vi "T1_Pulse_CommandSTR_gen.vi"(0 "T1 Pulse Sequence":T2={"Preliminary Settings"={"Nº of Scans (ns)"=3, "Pulse Frequency"=10000000.0, "Nº of Vd"=3}, "Pulse Settings"={"Duration Signal P2"=20.0, "Power Level P2"=1023, "Phase P2"=90, "P2 Unit"=0, "Duration Signal P1"=20.0, "Power Level P1"=1023, "Phase P1"=90, "P1 Unit"=0}, "Acquisition Settings"={"Number Samples"=2000, "Time Between Points"=0.0, "Unit"=0}, "Delay Settings"={"Delay d1"=10.0, "Delay d2"=0.0, "d1 Unit"=0, "d2 Unit"=0, "Delay d30"=0.0, "d30 Unit"=0, "Vd Unit"=0, "Vd Values"="1"}} {"Delay Settings"."Vd Unit" items=["us", "ms"]; "Delay Settings"."d30 Unit" items=["us", "ms"]; "Delay Settings"."Delay d30" min=0.0 step=1.0; "Delay Settings"."d2 Unit" items=["us", "ms"]; "Delay Settings"."d1 Unit" items=["us", "ms"]; "Delay Settings"."Delay d2" min=0.0 step=1.0 format="%#_4g"; "Delay Settings"."Delay d1" min=0.0 step=1.0 format="%#_4g"; "Acquisition Settings"."Unit" items=["us", "ms"]; "Acquisition Settings"."Time Between Points" min=0.0 step=1.0; "Acquisition Settings"."Number Samples" step=1; "Pulse Settings"."P1 Unit" items=["us", "ms"]; "Pulse Settings"."Phase P1" max=270 step=90; "Pulse Settings"."Power Level P1" max=1023 step=1; "Pulse Settings"."Duration Signal P1" min=0.0 step=1.0 format="%#_4g"; "Pulse Settings"."P2 Unit" items=["us", "ms"]; "Pulse Settings"."Phase P2" max=270 step=90; "Pulse Settings"."Power Level P2" max=1023 step=1; "Pulse Settings"."Duration Signal P2" min=0.0 step=1.0 format="%#_4g"; "Preliminary Settings"."Nº of Vd" step=1; "Preliminary Settings"."Pulse Frequency" min=1.0 max=200000000.0 step=1000000.0 format="%^#_6e"; "Preliminary Settings"."Nº of Scans (ns)" step=1}, 5 "Manual Vd":dbl[](array[numeric])=[10.0, 340.0, 670.0, 1000.0] min=1.0 step=1.0) -> (4 "Array":string[](array[string]), 6 "T1 set times":T1={"Real Time P1"=20.011287076734621636, "Real Time P2"=20.011287076734621636, "Real Time d1"=10.036661125207804438, "Real Time d2"=1.462, "Real Time d30"=1.462, "Real Time AQS"=0.73746299999999999998}, 12 "Values Vd Used":dbl[](array[numeric]))   [LabVIEW 2011]
uses:
  Controls/Full_T1 Degree Pulse Settings.ctl
  Controls/T1_Preliminary Settings.ctl
  Controls/T1_Pulse Settings.ctl
  Controls/Acquisition Settings.ctl
  Controls/T1_Delay Settings.ctl
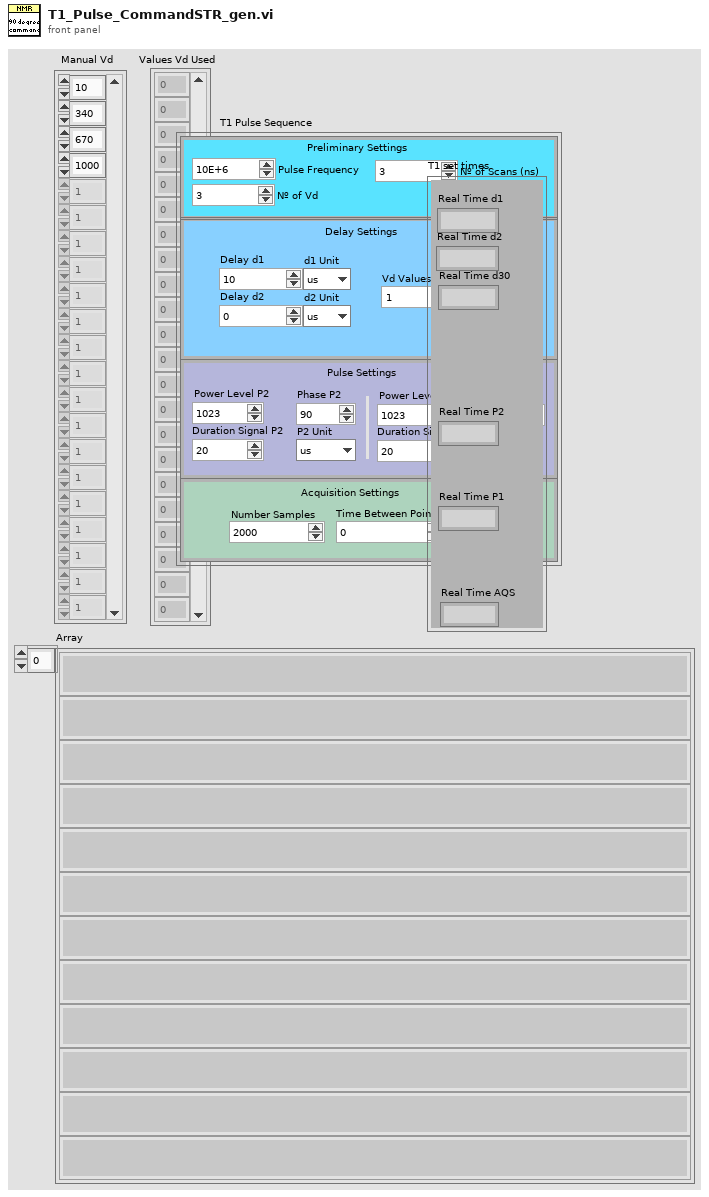
[diagram p1: front panel]
types:
  T1 = cluster{"Real Time P1":ext, "Real Time P2":ext, "Real Time d1":ext, "Real Time d2":ext, "Real Time d30":ext, "Real Time AQS":ext}
  T2 = typedef "Full_T1 Degree Pulse Settings.ctl" = cluster{"Preliminary Settings":T3, "Pulse Settings":T4, "Acquisition Settings":T5, "Delay Settings":T6}
  T3 = typedef "T1_Preliminary Settings.ctl" = cluster{"Nº of Scans (ns)":u16, "Pulse Frequency":dbl, "Nº of Vd":u16}
  T4 = typedef "T1_Pulse Settings.ctl" = cluster{"Duration Signal P2":dbl, "Power Level P2":u16, "Phase P2":u16, "P2 Unit":u8, "Duration Signal P1":dbl, "Power Level P1":u16, "Phase P1":u16, "P1 Unit":u8}
  T5 = typedef "Acquisition Settings.ctl" = cluster{"Number Samples":u16, "Time Between Points":dbl, "Unit":u8}
  T6 = typedef "T1_Delay Settings.ctl" = cluster{"Delay d1":dbl, "Delay d2":dbl, "d1 Unit":u8, "d2 Unit":u8, "Delay d30":dbl, "d30 Unit":u8, "Vd Unit":u8, "Vd Values":string}
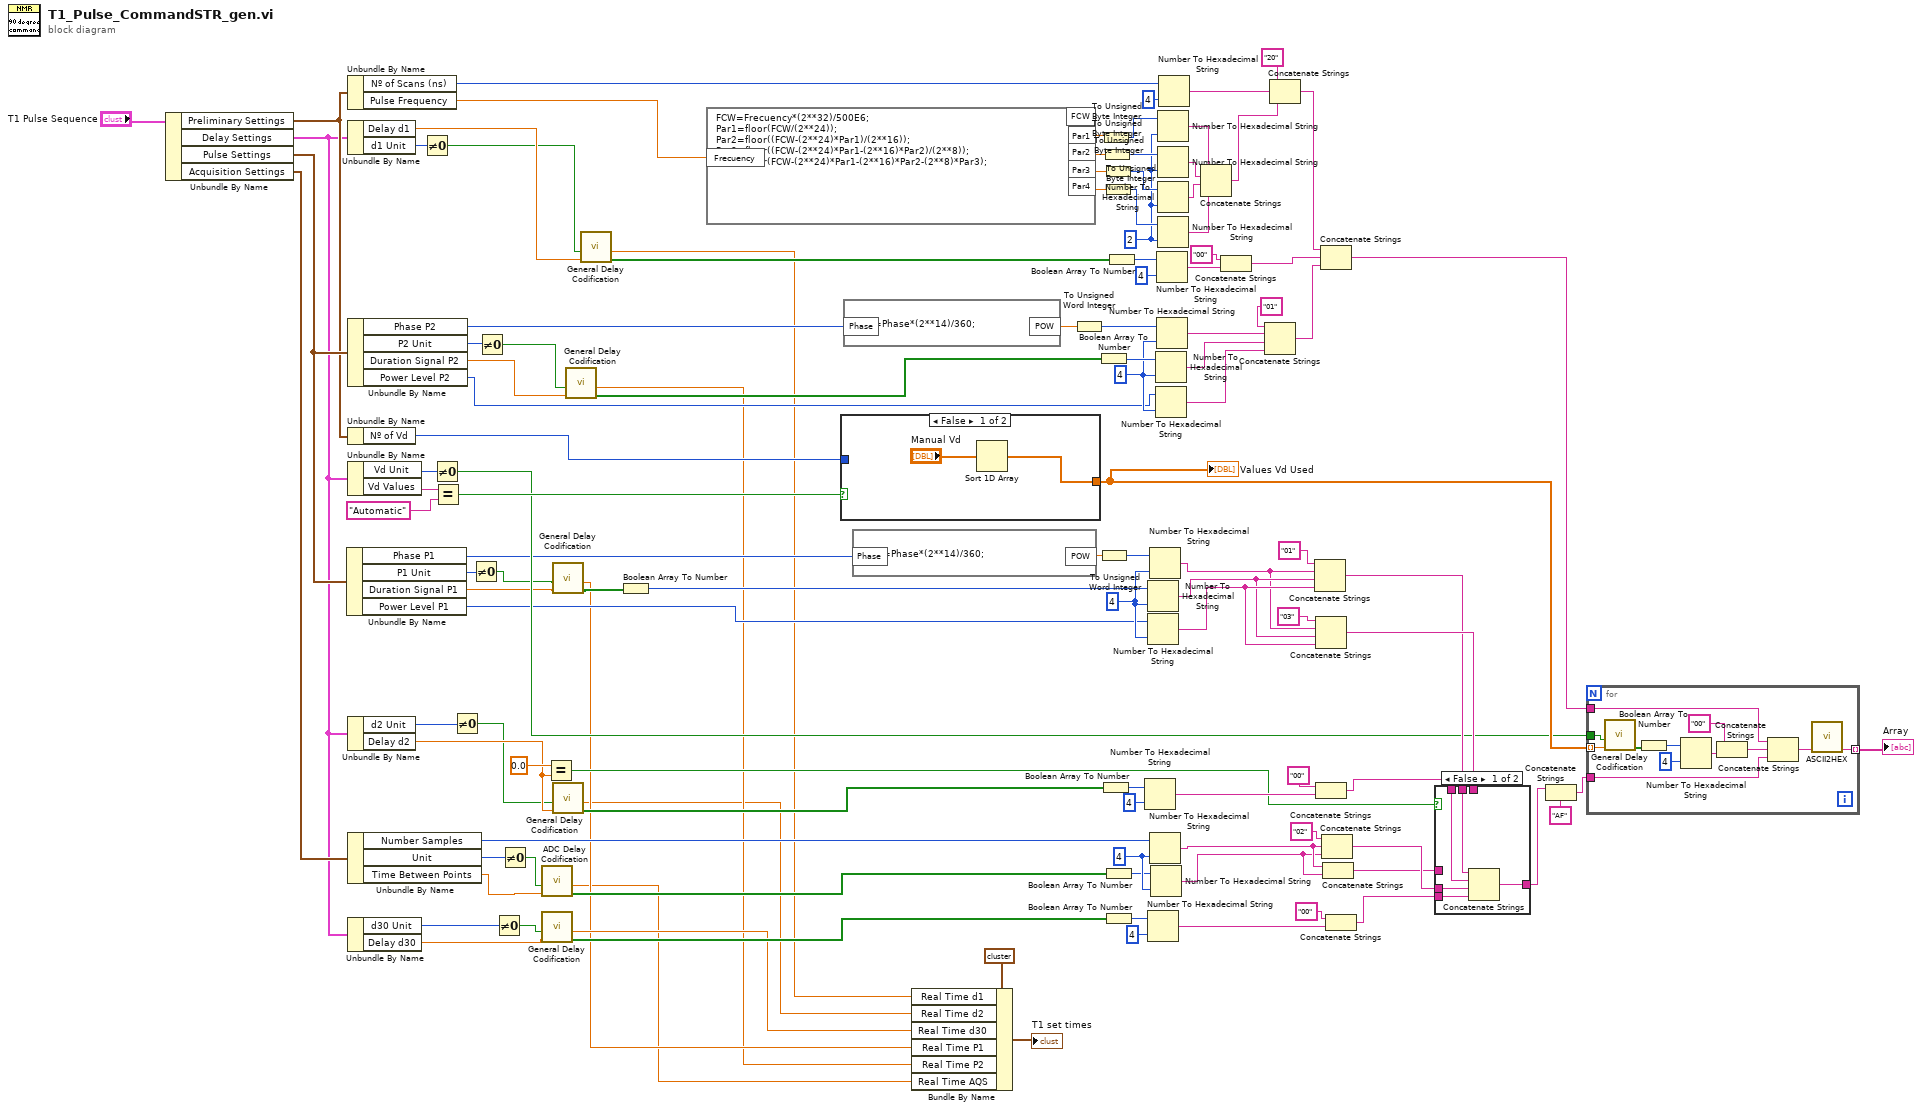
[diagram p0: block diagram]
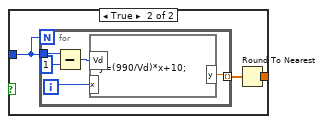
[diagram p2: hidden frame]
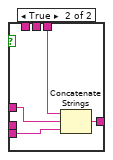
[diagram p3: hidden frame]
diagram:
  w78 = i16 2 ("width (-)")
  w106 = i16 4 ("width (-)")
  w55 = i16 4 ("width (-)")
  w56 = i16 4 ("width (-)")
  n1 = Unbundle By Name("T1 Pulse Sequence") -> ("Preliminary Settings"=w41:T3, "Delay Settings"=w27:T6, "Pulse Settings"=w45:T4, "Acquisition Settings"=w118:T5)
  n2 = Unbundle By Name(w45) -> ("Phase P1"=w32:u16, "P1 Unit"=w33:u8, "Duration Signal P1"=w20:dbl, "Power Level P1"=w34:u16)
  n3 = Unbundle By Name(w41) -> ("Nº of Scans (ns)"=w48:u16, "Pulse Frequency"=w47:dbl)
  n4 = Unbundle By Name(w27) -> ("Delay d1"=w14:dbl, "d1 Unit"=w46:u8)
  n5 = Unbundle By Name(w45) -> ("Phase P2"=w44:u16, "P2 Unit"=w43:u8, "Duration Signal P2"=w17:dbl, "Power Level P2"=w42:u16)
  n6 = Unbundle By Name(w41) -> ("Nº of Vd"=w40:u16)
  n7 = Unbundle By Name(w27) -> ("Vd Unit"=w36:u8, "Vd Values"=w39:string)
  n8 = Unbundle By Name(w27) -> ("d2 Unit"=w29:u8, "Delay d2"=w23:dbl)
  n9 = Unbundle By Name(w118) -> ("Number Samples"=w31:u16, "Unit"=w28:u8, "Time Between Points"=w9:dbl)
  n10 = Unbundle By Name(w27) -> ("d30 Unit"=w30:u8, "Delay d30"=w25:dbl)
  n11 = Not Equal To 0?(x=w46) -> (x != 0?=w13:bool)
  n12 = Not Equal To 0?(x=w36) -> (x != 0?=w35:bool)
  n13 = Equal?(x=w39, y="Automatic") -> (x = y?=w37:bool)
  n14 = Not Equal To 0?(x=w29) -> (x != 0?=w22:bool)
  n15 = Not Equal To 0?(x=w33) -> (x != 0?=w19:bool)
  n16 = Not Equal To 0?(x=w43) -> (x != 0?=w15:bool)
  n17 = Not Equal To 0?(x=w30) -> (x != 0?=w26:bool)
  n18 = Not Equal To 0?(x=w28) -> (x != 0?=w10:bool)
  n19 = call "ADC Delay Codification.vi"("Delay"=w9, "ms/us Delay"=w10) -> ("Final array"=w11:bool[], "Real Time"=w3:ext)  [unwired: 8 in]
  n20 = call "General Delay Codification.vi"("Delay"=w25, "ms/us Delay"=w26) -> ("Final array"=w24:bool[], "Real Time"=w6:ext)  [unwired: 8 in]
  n21 = Equal?(x=0.0 ("y"), y=w23) -> (x = y?=w65:bool)
  n22 = call "General Delay Codification.vi"("Delay"=w20, "ms/us Delay"=w19) -> ("Final array"=w18:bool[], "Real Time"=w5:ext)  [unwired: 8 in]
  n23 = call "General Delay Codification.vi"("Delay"=w23, "ms/us Delay"=w22) -> ("Final array"=w21:bool[], "Real Time"=w1:ext)  [unwired: 8 in]
  n24 = call "General Delay Codification.vi"("Delay"=w17, "ms/us Delay"=w15) -> ("Final array"=w16:bool[], "Real Time"=w4:ext)  [unwired: 8 in]
  n25 = call "General Delay Codification.vi"("Delay"=w14, "ms/us Delay"=w13) -> ("Final array"=w12:bool[], "Real Time"=w7:ext)  [unwired: 8 in]
  n26 = Boolean Array To Number(Boolean array=w18) -> (number=w90:u32)
  n27 = formula code="FCW=Frecuency*(2**32)/500E6;\nPar1=floor(FCW/(2**24));\nPar2=floor((FCW-(2**24)*Par1)/(2**16));\nPar3=floor((FCW-(2**24)*Par1-(2**16)*Par2)/(2**8));\nPar4=floor(FCW-(2**24)*Par1-(2**16)*Par2-(2**8)*Par3);"("Frecuency"=w47) -> ("Par1"=w82:dbl, "Par2"=w81:dbl, "Par3"=w80:dbl, "Par4"=w79:dbl)  [unwired: 1 out]
  n28 = case shown="False" w37 {
    tunnel: [w120 w123] -> w50
    tunnel: w40 -> [_ w121]
    frame False {
      n29 = Sort 1D Array(array="Manual Vd") -> (sorted array=w120:dbl[])
    }
    frame True {
      n30 = for {
        N: w121 -> [_]
        tunnel: w121 -> [w126]
        tunnel: [w127] -> w122 mode=indexing
        i -> [w128]
        n31 = Subtract(x=w126, y=u8 1) -> (x-y=w124:u16)
        n32 = formula code="y=(990/Vd)*x+10;"("x"=w128, "Vd"=w124) -> ("y"=w127:dbl)
      }
      n33 = Round To Nearest(number=w122) -> (nearest integer value=w123:dbl[])
    }
  }
  "Values Vd Used" <- w50
  n34 = formula code="POW=Phase*(2**14)/360;"("Phase"=w44) -> ("POW"=w72:dbl)
  n35 = formula code="POW=Phase*(2**14)/360;"("Phase"=w32) -> ("POW"=w67:dbl)
  n36 = Bundle By Name(cluster=T1 {"Real Time P1"=0.0, "Real Time P2"=0.0, "Real Time d1"=0.0, "Real Time d2"=0.0, "Real Time d30"=0.0, "Real Time AQS"=0.0} ("Cluster 2"), "Real Time d1"=w7, "Real Time d2"=w1, "Real Time d30"=w6, "Real Time P1"=w5, "Real Time P2"=w4, "Real Time AQS"=w3) -> (→"T1 set times":T1)
  n37 = To Unsigned Word Integer(number=w72) -> (unsigned 16bit integer=w71:u16)
  n38 = Boolean Array To Number(Boolean array=w16) -> (number=w92:u32)
  n39 = To Unsigned Word Integer(number=w67) -> (unsigned 16bit integer=w66:u16)
  n40 = To Unsigned Byte Integer(number=w82) -> (unsigned 8bit integer=w86:u8)
  n41 = Boolean Array To Number(Boolean array=w21) -> (number=w91:u32)
  n42 = To Unsigned Byte Integer(number=w81) -> (unsigned 8bit integer=w85:u8)
  n43 = To Unsigned Byte Integer(number=w80) -> (unsigned 8bit integer=w84:u8)
  n44 = To Unsigned Byte Integer(number=w79) -> (unsigned 8bit integer=w83:u8)
  n45 = Boolean Array To Number(Boolean array=w11) -> (number=w88:u32)
  n46 = Boolean Array To Number(Boolean array=w24) -> (number=w89:u32)
  n47 = Boolean Array To Number(Boolean array=w12) -> (number=w93:u32)
  n48 = Number To Hexadecimal String(1:i16 4 ("width (-)"), 2:w91) -> (0:w108:string)
  n49 = Number To Hexadecimal String(1:w55, 2:w90) -> (0:w63:string)
  n50 = Number To Hexadecimal String(1:w55, 2:w34) -> (0:w64:string)
  n51 = Number To Hexadecimal String(1:i16 4 ("width (-)"), 2:w89) -> (0:w103:string)
  n52 = Number To Hexadecimal String(1:w55, 2:w66) -> (0:w62:string)
  n53 = Number To Hexadecimal String(1:w106, 2:w31) -> (0:w59:string)
  n54 = Number To Hexadecimal String(1:w106, 2:w88) -> (0:w58:string)
  n55 = Number To Hexadecimal String(1:w56, 2:w92) -> (0:w69:string)
  n56 = Number To Hexadecimal String(1:w56, 2:w42) -> (0:w68:string)
  n57 = Number To Hexadecimal String(1:i16 4 ("width (-)"), 2:w93) -> (0:w113:string)
  n58 = Number To Hexadecimal String(1:w56, 2:w71) -> (0:w70:string)
  n59 = Number To Hexadecimal String(1:w78, 2:w86) -> (0:w77:string)
  n60 = Number To Hexadecimal String(1:w78, 2:w85) -> (0:w76:string)
  n61 = Number To Hexadecimal String(1:w78, 2:w84) -> (0:w75:string)
  n62 = Number To Hexadecimal String(1:w78, 2:w83) -> (0:w74:string)
  n63 = Number To Hexadecimal String(1:i16 4 ("width (-)"), 2:w48) -> (0:w101:string)
  n64 = Concatenate Strings(w77, w76, w75, w74) -> (w73:string)
  n65 = Concatenate Strings("00" ("string"), w113) -> (w98:string)
  n66 = Concatenate Strings("01" ("string"), w70, w69, w68) -> (w97:string)
  n67 = Concatenate Strings("20" ("string"), w101, w73) -> (w99:string)
  n68 = Concatenate Strings("01" ("string"), w62, w63, w64) -> (w52:string)
  n69 = Concatenate Strings("03" ("string"), w62, w63, w64) -> (w60:string)
  n70 = Concatenate Strings("00" ("string"), w108) -> (w96:string)
  n71 = Concatenate Strings(w99, w98, w97) -> (w51:string)
  n72 = Concatenate Strings("02" ("string"), w59, w58) -> (w95:string)
  n73 = Concatenate Strings(w59, w58) -> (w57:string)
  n74 = Concatenate Strings("00" ("string"), w103) -> (w54:string)
  n75 = case shown="False" w65 {
    tunnel: w96 -> [w133 _]
    tunnel: w95 -> [w132 _]
    tunnel: [w131 w137] -> w94
    tunnel: w54 -> [w130 w135]
    tunnel: w52 -> [w129 _]
    tunnel: w60 -> [_ w136]
    tunnel: w57 -> [_ w134]
    frame False {
      n76 = Concatenate Strings(w129, w133, w132, w130) -> (w131:string)
    }
    frame True {
      n77 = Concatenate Strings(w136, w134, w135) -> (w137:string)
    }
  }
  n78 = Concatenate Strings(w94, "AF" ("string")) -> (w49:string)
  n79 = for {
    tunnel: w49 -> [w143]
    tunnel: w50 -> [w140] mode=indexing
    tunnel: w51 -> [w144]
    tunnel: w35 -> [w139]
    tunnel: [w141] -> w116 mode=indexing
    n80 = call "General Delay Codification.vi"("Delay"=w140, "ms/us Delay"=w139) -> ("Final array"=w138:bool[])  [unwired: 8 in, 1 out]
    n81 = Boolean Array To Number(Boolean array=w138) -> (number=w148:u32)
    n82 = Number To Hexadecimal String(1:i16 4 ("width (-)"), 2:w148) -> (0:w147:string)
    n83 = Concatenate Strings("00" ("string"), w147) -> (w145:string)
    n84 = Concatenate Strings(w144, w145, w143) -> (w142:string)
    n85 = call "ASCII2HEX.vi"("String (Normal Display)"=w142) -> ("Result string (Hex Display)"=w141:string)  [unwired: 10 in]
  }
  "Array" <- w116
